vi "Change Color.vi"(8 "error in (no error)":errorcluster, 10 "Status":T1[](array[typedef]), 11 "AllObjs[]":refnum<vi>[](array[refnum])) -> (0 "error out":errorcluster)   [LabVIEW 2013]
uses:
  Controls/Security Zones.ctl
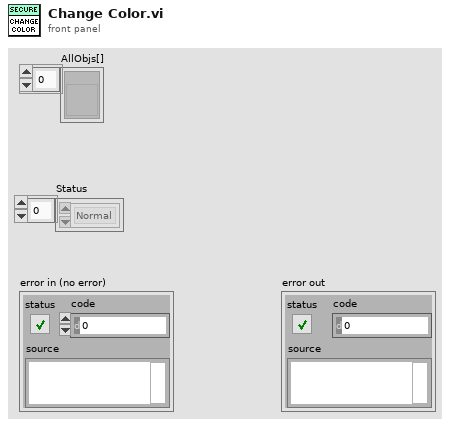
[diagram p1: front panel]
types:
  T1 = typedef "Security Zones.ctl" = enum16{"Normal", "Alarm", "Bypass", "Tamper"}
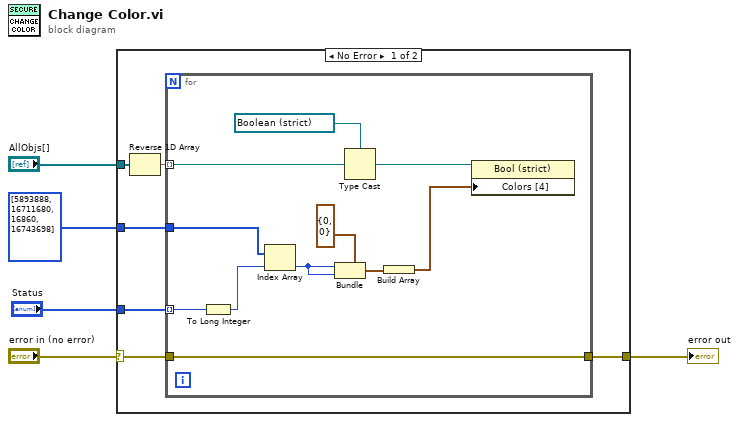
[diagram p0: block diagram]
diagram:
  n1 = case shown="No Error" "error in (no error)" {
    selector: "error in (no error)" -> [w7 w23]
    tunnel: "AllObjs[]" -> [w11 _]
    tunnel: "Status" -> [w10 _]
    tunnel: [w8 w23] -> w5
    tunnel: u32[] [5893888, 16711680, 16860, 16743698] -> [w6 _]
    frame No Error {
      n2 = Reverse 1D Array(array=w11) -> (reversed array=w9:refnum<vi>[])
      n3 = for {
        tunnel: w10 -> [w22] mode=indexing
        tunnel: w9 -> [w21] mode=indexing
        tunnel: [w14] -> w8
        tunnel: w7 -> [w14]
        tunnel: w6 -> [w13]
        n4 = To Long Integer(number=w22) -> (32bit integer=w12:i32)
        n5 = Index Array(array=w13, index=w12) -> (element=w17:u32)
        n6 = Bundle(cluster=cluster{u32, u32} {0, 0}, w17, w17) -> (w16:cluster{u32, u32})
        n7 = Type Cast(type=refnum<vi> refnum ("reference"), x=w21) -> (*(type *) &x=w20:refnum<vi>)
        n8 = Build Array(w16) -> (w15:cluster{u32, u32}[])
        n9 = property on="Property Node" class="Bool (strict)"(reference=w20, "Colors [4]"=w15) -> ()  [unwired: 1 in, 2 out]
      }
    }
    frame Error {
    }
  }
  "error out" <- w5
